vi "Pack Step Value.vi"(8 "error in (no error)":errorcluster, 10 "Value":string, 11 "Wait STEP in":refnum<class "Wait STEP.lvclass">=refnum) -> (0 "error out":errorcluster, 3 "Wait STEP out":refnum<class "Wait STEP.lvclass">)   [LabVIEW 2014, in "Wait STEP.lvlib" / "Wait STEP.lvclass"]
uses:
  Wait STEP.lvclass
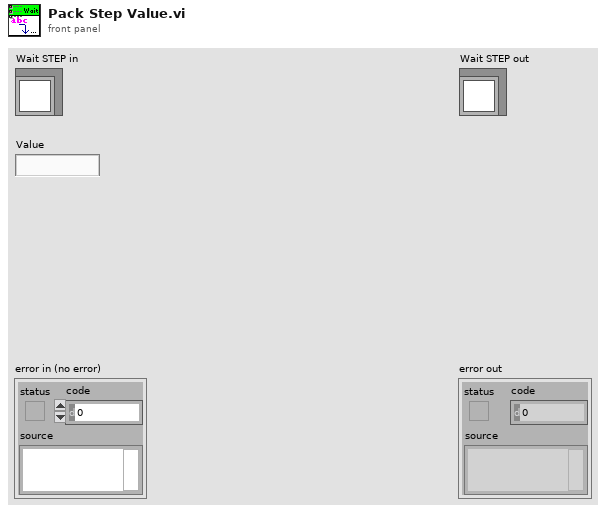
[diagram p1: front panel]
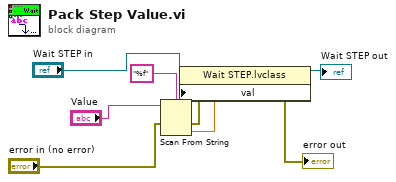
[diagram p0: block diagram]
diagram:
  n1 = Scan From String(format string="%f", input string="Value", error in="error in (no error)") -> (error out=w2:errorcluster, output 1=w3:dbl)  [unwired: 2 in, 2 out]
  n2 = property class="Wait STEP.lvclass"(reference="Wait STEP in", error in=w2, "val"=w3) -> (reference out=→"Wait STEP out":refnum<class "Wait STEP.lvclass">, error out=→"error out":errorcluster)
